vi "WinCI File History.vi"(6 "versions":string[](array[string]), 7 "advanced options":variant, 8 "error in (no error)":errorcluster, 10 "files":path[](array[path]), 11 "source control reference in":T1) -> (0 "error out":errorcluster, 2 "status message":string, 3 "source control reference out":T1, 5 "file changed?":bool)   [LabVIEW 2020, in "NI_SCC_WinCI.lvlib"]
uses:
  <vilib>/SourceControl/Providers/WinCI/NI_SCC_WinCI.lvlib
  <vilib>/SourceControl/sccapi/SCCAPI Refnum.ctl
  <vilib>/SourceControl/support/SCCSup Message Strings GLBL.vi
  <vilib>/SourceControl/sccapi/NI_SCC.lvlib
panel:
  out "result":i32
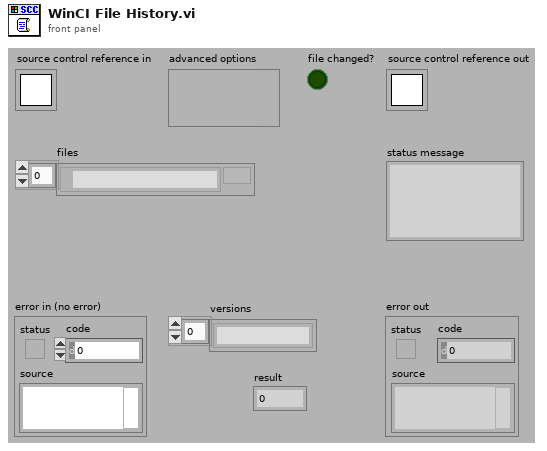
[diagram p1: front panel]
types:
  T1 = typedef "NI_SCC.lvlib/SCCAPI Refnum.ctl" = refnum<k1>
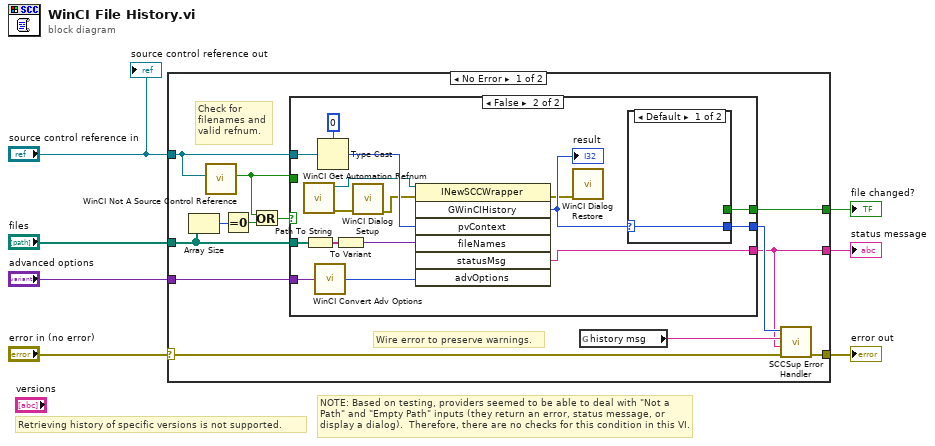
[diagram p0: block diagram]
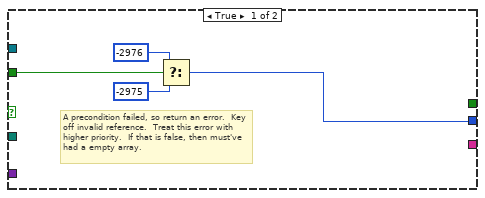
[diagram p2: hidden frame]
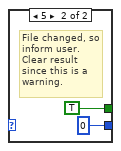
[diagram p3: hidden frame]
diagram:
  # "NOTE: Based on testing, providers seemed to be able to deal with \"Not a Path\" and \"Empty Path\" inputs (they return an error, status message, or display a dialog).  Therefore, there are no checks for this condition in this VI."
  # "Retrieving history of specific versions is not supported."
  n1 = case shown="No Error" "error in (no error)" {
    selector: "error in (no error)" -> [w12 w44]
    tunnel: [w19 w44] -> w6
    tunnel: "source control reference in" -> [w9 _]
    tunnel: [w16 _] -> w4
    tunnel: "files" -> [w20 _]
    tunnel: [w11 _] -> w2
    tunnel: "advanced options" -> [w10 _]
    frame No Error {
      # "Wire error to preserve warnings."
      # "Check for filenames and valid refnum."
      n2 = Array Size(array=w20) -> (size(s)=w15:i32)
      n3 = call <vilib>:"WinCI Not A Source Control Reference.vi"("source control reference in"=w9) -> ("not a source control reference?"=w8:bool)  [unwired: 1 in, 9 out]
      n4 = Equal To 0?(x=w15) -> (x = 0?=w14:bool)
      n5 = Or(x=w8, y=w14) -> (x .or. y?=w13:bool)
      n6 = case shown="False" w13 {
        tunnel: w9 -> [_ w40]
        tunnel: [_ w30] -> w16
        tunnel: w20 -> [_ w38]
        tunnel: [w21 w37] -> w18
        tunnel: w8 -> [w22 _]
        tunnel: [_ w36] -> w11
        tunnel: w10 -> [_ w35]
        frame True {
          # "A precondition failed, so return an error.  Key off invalid reference.  Treat this error with higher priority.  If that is false, then must've had a empty array."
          n7 = Select(t=-2976 ("result"), s=w22, f=-2975 ("result")) -> (s? t:f=w21:i32)
        }
        frame False {
          n8 = call <vilib>:"WinCI Get Automation Refnum.vi"() -> ("error out"=w27:errorcluster, "automation refnum"=w28:refnum<k7>)  [unwired: 10 out]
          n9 = Path To String(path=w38) -> (string=w34:string[])
          n10 = call <vilib>:"WinCI Convert Adv Options.vi"("advanced options"=w35) -> ("command options"=w32:u32)  [unwired: 4 out]
          n11 = Type Cast(type=u32 0, x=w40) -> (*(type *) &x=w31:u32)
          n12 = To Variant(anything=w34) -> (Variant=w33:variant)
          n13 = call <vilib>:"WinCI Dialog Setup.vi"("error in"=w27) -> ("error out"=w26:errorcluster)  [unwired: 10 out]
          n14 = invoke class="INewSCCWrapper" method="GWinCIHistory"(reference=w28, error in=w26, "pvContext"=w31, "fileNames"=w33, "advOptions"=w32) -> (error out=w25:errorcluster, "GWinCIHistory"=w29:i32, "statusMsg"=w30:string)  [unwired: 2 in, 4 out]
          "result" <- w29
          n15 = call <vilib>:"WinCI Dialog Restore.vi"("error in"=w25) -> ()  [unwired: 11 out]
          n16 = case shown="Default" w29 {
            selector: w29 -> [w41 _]
            tunnel: [w41 0 ("result")] -> w37
            tunnel: [_ TRUE] -> w36
            frame Default {
            }
            frame 5 {
              # "File changed, so inform user.  Clear result since this is a warning."
            }
          }
        }
      }
      n17 = global read "SCCSup Message Strings GLBL.vi" "history msg"() -> (w17:string)
      n18 = call <vilib>:"SCCSup Error Handler.vi"("error in (no error)"=w12, "additional message"=w16, "operation message"=w17, "scc error code"=w18) -> ("error out"=w19:errorcluster)  [unwired: 7 out]
    }
    frame Error {
    }
  }
  "error out" <- w6
  "status message" <- w4
  "file changed?" <- w2
  "source control reference out" <- "source control reference in"
